vi "extractNamedChildXML.vi"(8 "error in (no error)":errorcluster, 10 "childName":string, 11 "ReadElement in":refnum<class "XMLParser.lvclass">) -> (0 "error out":errorcluster, 1 "ChildContentsEmpty":bool, 2 "childXML":string, 3 "ReadElement out":refnum<class "XMLParser.lvclass">)   [LabVIEW 2016, in "XML.lvlib" / "XMLParser.lvclass"]
doc: "Extracts the child XML and its contents as determined by the childName input."
uses:
  <userlib>/Common/XML/XMLParser/XMLParser.lvclass
  <userlib>/Common/XML/XMLParser/XMLParser.lvclass/XMLParser.ctl
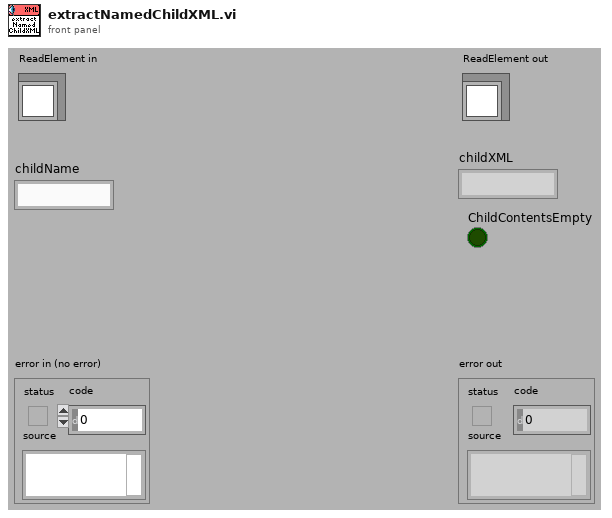
[diagram p1: front panel]
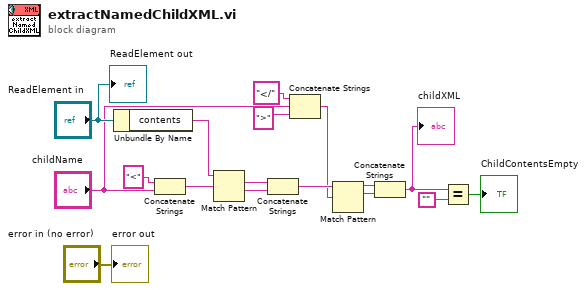
[diagram p0: block diagram]
diagram:
  n1 = Unbundle By Name("ReadElement in") -> ("contents"=w5:string)
  n2 = Concatenate Strings("<" ("string"), "childName") -> (w14:string)
  n3 = Match Pattern(string=w5, regular expression=w14) -> (match substring=w11:string, after substring=w10:string)  [unwired: 1 in, 2 out]
  n4 = Concatenate Strings(w11, w10) -> (w9:string)
  n5 = Concatenate Strings("</" ("string"), "childName", ">" ("string")) -> (w8:string)
  n6 = Match Pattern(string=w9, regular expression=w8) -> (before substring=w7:string, match substring=w6:string)  [unwired: 1 in, 2 out]
  n7 = Concatenate Strings(w7, w6) -> (w1:string)
  "childXML" <- w1
  n8 = Equal?(x=w1, y="") -> (x = y?=→"ChildContentsEmpty":bool)
  "error out" <- "error in (no error)"
  "ReadElement out" <- "ReadElement in"
